vi "IO Nodes Close References.vi"(8 "error in (no error)":errorcluster, 10 "Virtual Folder":refnum<vi>, 11 "Project in":refnum<vi>) -> (0 "error out":errorcluster)   [LabVIEW 2014, in "SPI Engine Scripting.lvlib"]
uses:
  SPI Engine Scripting.lvlib
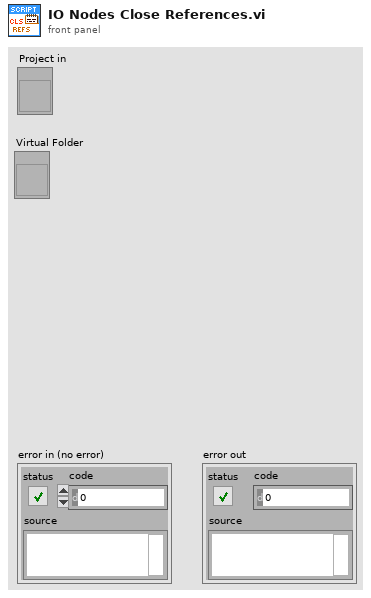
[diagram p1: front panel]
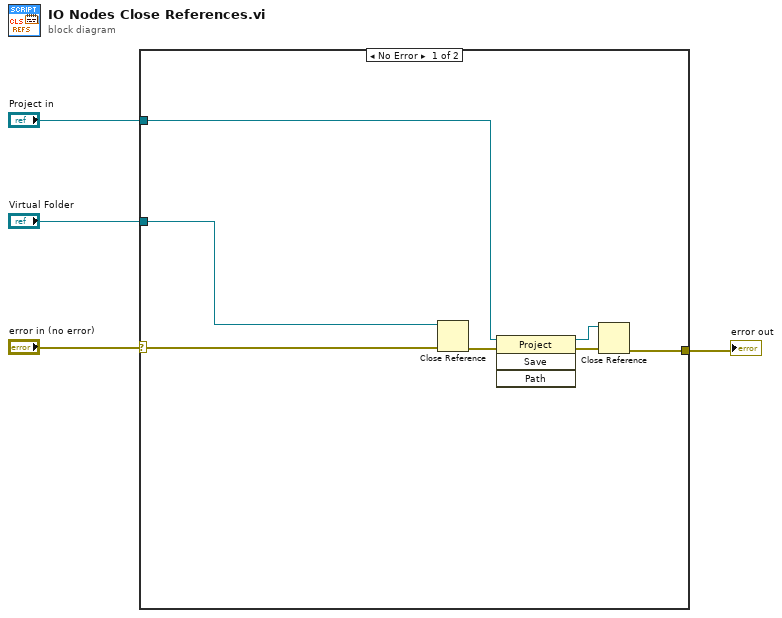
[diagram p0: block diagram]
diagram:
  n1 = case shown="No Error" "error in (no error)" {
    selector: "error in (no error)" -> [w5 w12]
    tunnel: "Project in" -> [w9 _]
    tunnel: [w11 w12] -> w4
    tunnel: "Virtual Folder" -> [w6 _]
    frame No Error {
      n2 = Close Reference(reference=w6, error in (no error)=w5) -> (error out=w10:errorcluster)
      n3 = invoke class="Project" method="Save"(reference=w9, error in=w10) -> (reference out=w8:refnum<vi>, error out=w7:errorcluster)  [unwired: 2 in, 2 out]
      n4 = Close Reference(reference=w8, error in (no error)=w7) -> (error out=w11:errorcluster)
    }
    frame Error {
    }
  }
  "error out" <- w4
